vi "bigcryo_H-control.vi"(9 "Rate [T/min]":dbl=0.5, 10 "Set Field [T]":dbl, 11 "Magnet Power supply":refnum<visa-resource-name>="COM6") -> ()   [LabVIEW 2019]
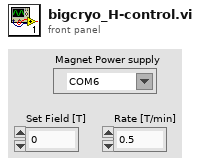
[diagram p1: front panel]
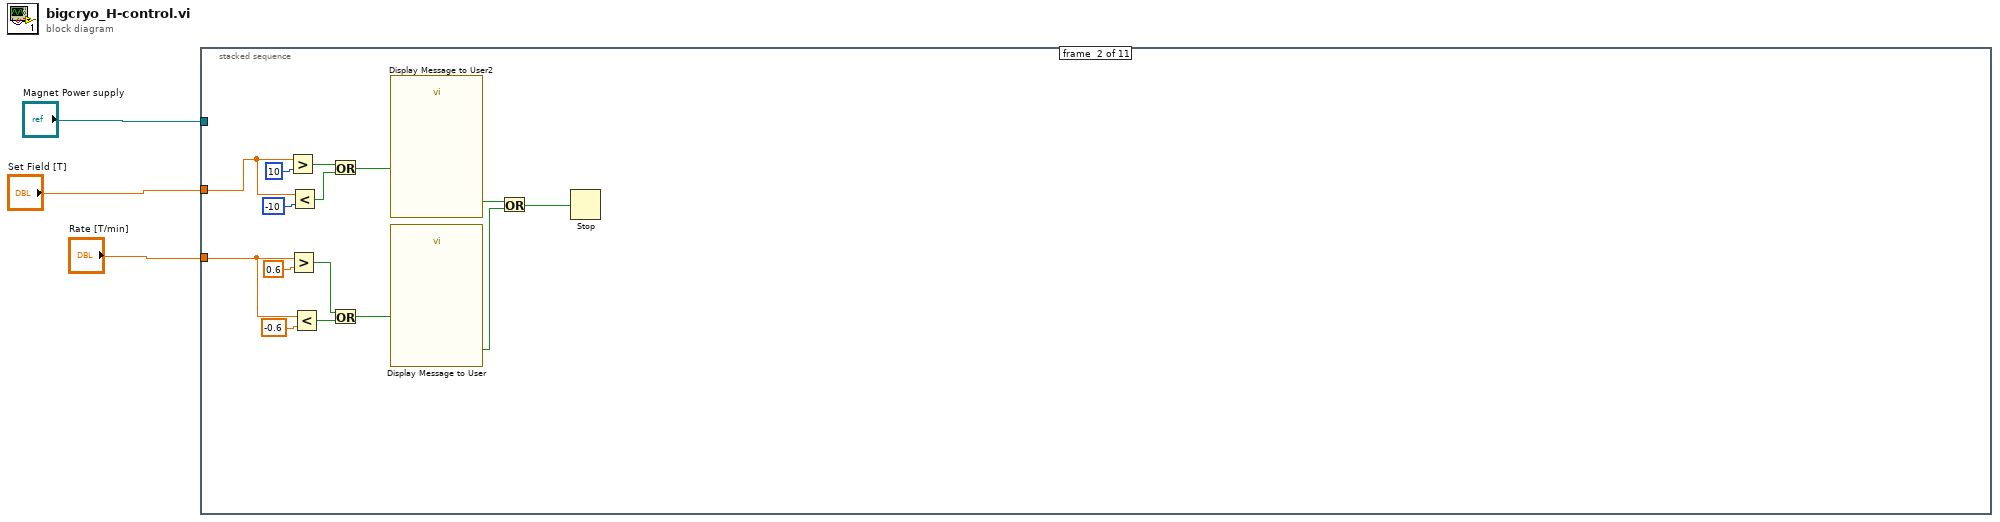
[diagram p0: block diagram]
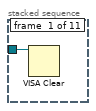
[diagram p2: hidden frame]
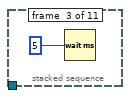
[diagram p3: hidden frame]
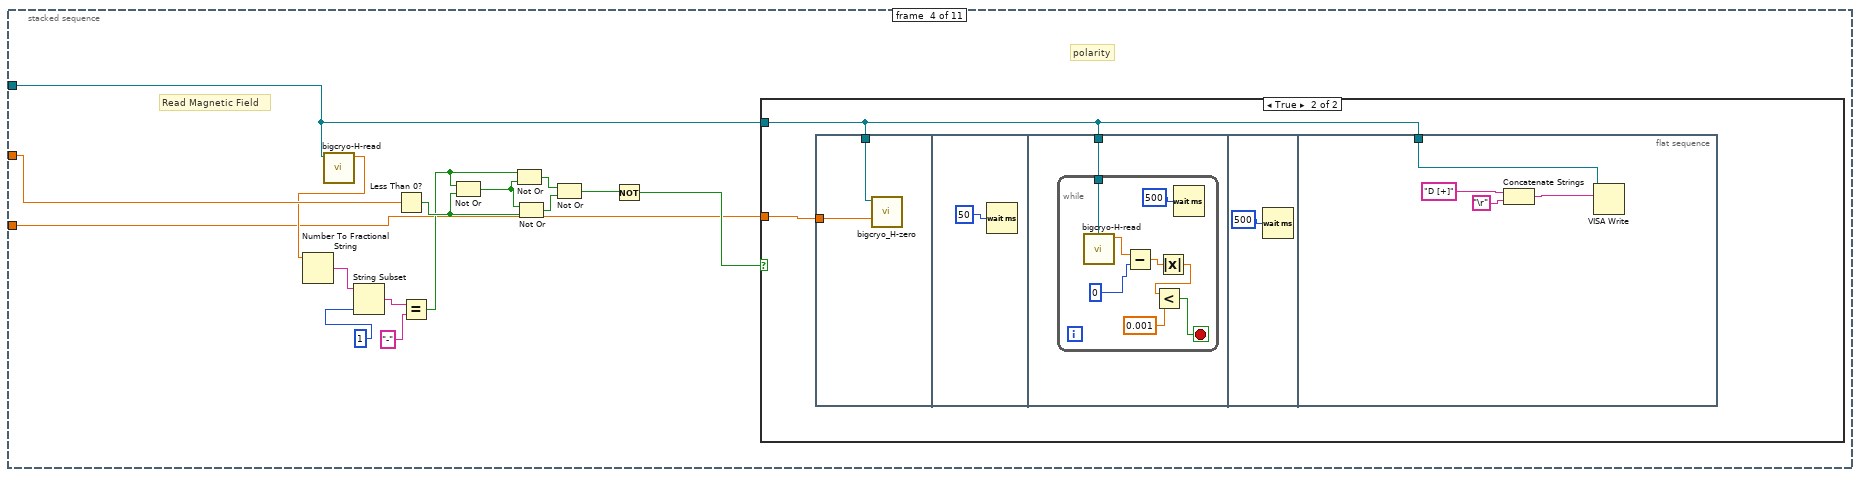
[diagram p4: hidden frame]
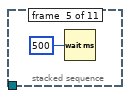
[diagram p6: hidden frame]
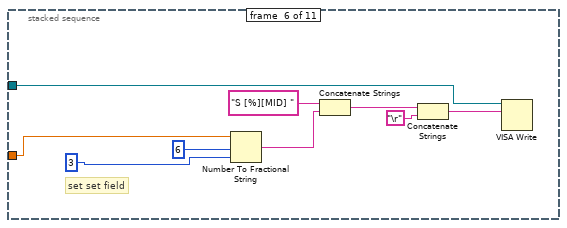
[diagram p7: hidden frame]
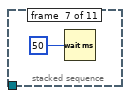
[diagram p8: hidden frame]
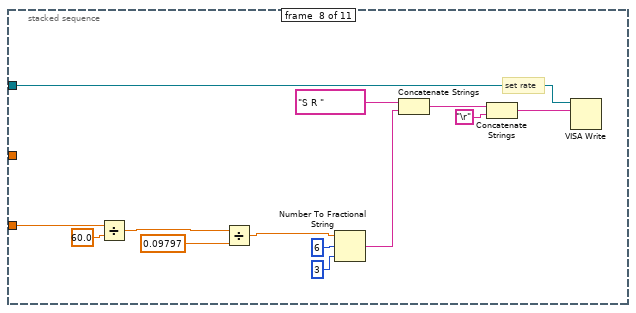
[diagram p9: hidden frame]
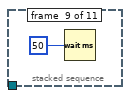
[diagram p10: hidden frame]
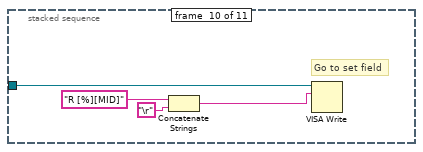
[diagram p11: hidden frame]
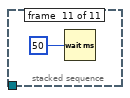
[diagram p12: hidden frame]
diagram:
  n1 = stacked-sequence {
    tunnel: "Magnet Power supply" -> [w4 _ _ w35 _ w58 _ w76 _ w81 _]
    tunnel: "Rate [T/min]" -> [_ w6 _ w21 _ _ _ w66 _ _ _]
    tunnel: "Set Field [T]" -> [_ w5 _ w34 _ w56 _ _ _ _ _]
    frame #0 {
      n2 = VISA Clear(VISA resource name=w4) -> ()  [unwired: 1 in, 2 out]
    }
    frame #1 {
      n3 = Greater?(x=w5, y=10) -> (0:w7:bool)
      n4 = Greater?(x=w6, y=0.6) -> (0:w16:bool)
      n5 = Less?(x=w5, y=-10) -> (x < y?=w12:bool)
      n6 = Less?(x=w6, y=-0.6) -> (x < y?=w15:bool)
      n7 = Or(x=w7, y=w12) -> (x .or. y?=w18:bool)
      n8 = Or(x=w16, y=w15) -> (x .or. y?=w17:bool)
      n9 = call "Display Message to User2"("Enable"=w18) -> ("OK"=w19:bool)  [unwired: 9 in, 1 out]
      n10 = call "Display Message to User"("Enable"=w17) -> ("OK"=w8:bool)  [unwired: 9 in, 1 out]
      n11 = Or(x=w19, y=w8) -> (x .or. y?=w9:bool)
      n12 = Stop(stop? (T)=w9) -> ()
    }
    frame #2 {
      n13 = Wait (ms)(milliseconds to wait=5) -> ()  [unwired: 1 out]
    }
    frame #3 {
      # "Read Magnetic Field"
      # "polarity"
      n14 = call "bigcryo-H-read.vi"("Magnet Power supply"=w35) -> ("Magnetic Field [T]"=w23:dbl)  [unwired: 9 in, 1 out]
      n15 = Number To Fractional String(number=w23) -> (F-format string=w26:string)  [unwired: 3 in]
      n16 = String Subset(string=w26, length (rest)=1 ("length (rest)")) -> (substring=w25:string)  [unwired: 1 in]
      n17 = Less Than 0?(x=w34) -> (x < 0?=w33:bool)
      n18 = Equal?(x=w25, y="-") -> (x = y?=w22:bool)
      n19 = Not Or(1:w33, 2:w22) -> (0:w32:bool)
      n20 = Not Or(1:w32, 2:w22) -> (0:w31:bool)
      n21 = Not Or(1:w33, 2:w32) -> (0:w30:bool)
      n22 = Not Or(1:w30, 2:w31) -> (0:w29:bool)
      n23 = Not(x=w29) -> (.not. x?=w28:bool)
      n24 = case shown="True" w28 {
        tunnel: w35 -> [_ w36]
        tunnel: w21 -> [_ w37]
        frame False {
        }
        frame True {
          n25 = flat-sequence {
            tunnel: w37 -> [w39]
            tunnel: w36 -> [w38]
            tunnel: w36 -> [w41]
            tunnel: w36 -> [w52]
            frame #0 {
              n26 = call "bigcryo_H-zero.vi"("Rate [T/min]"=w39, "Magnet Power supply"=w38) -> ()  [unwired: 10 in]
            }
            frame #1 {
              n27 = Wait (ms)(milliseconds to wait=50) -> ()  [unwired: 1 out]
            }
            frame #2 {
              n28 = while {
                tunnel: w41 -> [w49]
                stop <- w48 stop-if-true
                n29 = call "bigcryo-H-read.vi"("Magnet Power supply"=w49) -> ("Magnetic Field [T]"=w46:dbl)  [unwired: 9 in, 1 out]
                n30 = Subtract(x=w46, y=0) -> (x-y=w44:dbl)
                n31 = Absolute Value(x=w44) -> (abs(x)=w43:dbl)
                n32 = Less?(x=w43, y=0.001) -> (x < y?=w48:bool)
                n33 = Wait (ms)(milliseconds to wait=500) -> ()  [unwired: 1 out]
              }
            }
            frame #3 {
              n34 = Wait (ms)(milliseconds to wait=500) -> ()  [unwired: 1 out]
            }
            frame #4 {
              n35 = Concatenate Strings("D [+]" ("data"), "\r") -> (w54:string)
              n36 = VISA Write(VISA resource name=w52, write buffer=w54) -> ()  [unwired: 1 in, 3 out]
            }
          }
        }
      }
    }
    frame #4 {
      n37 = Wait (ms)(milliseconds to wait=500) -> ()  [unwired: 1 out]
    }
    frame #5 {
      # "set set field"
      n38 = Number To Fractional String(number=w56, width (-)=i16 6, precision (6)=i16 3) -> (F-format string=w61:string)  [unwired: 1 in]
      n39 = Concatenate Strings("S [%][MID] " ("string"), w61) -> (w57:string)
      n40 = Concatenate Strings(w57, "\r") -> (w60:string)
      n41 = VISA Write(VISA resource name=w58, write buffer=w60) -> ()  [unwired: 1 in, 3 out]
    }
    frame #6 {
      n42 = Wait (ms)(milliseconds to wait=50) -> ()  [unwired: 1 out]
    }
    frame #7 {
      # "set rate"
      n43 = Divide(x=w66, y=60.0) -> (x/y=w71:dbl)
      n44 = Divide(x=w71, y=0.09797) -> (x/y=w69:dbl)
      n45 = Number To Fractional String(number=w69, width (-)=i16 6, precision (6)=i16 3) -> (F-format string=w74:string)  [unwired: 1 in]
      n46 = Concatenate Strings("S R " ("string"), w74) -> (w73:string)
      n47 = Concatenate Strings(w73, "\r") -> (w78:string)
      n48 = VISA Write(VISA resource name=w76, write buffer=w78) -> ()  [unwired: 1 in, 3 out]
    }
    frame #8 {
      n49 = Wait (ms)(milliseconds to wait=50) -> ()  [unwired: 1 out]
    }
    frame #9 {
      # "Go to set field"
      n50 = Concatenate Strings("R [%][MID]" ("data"), "\r") -> (w83:string)
      n51 = VISA Write(VISA resource name=w81, write buffer=w83) -> ()  [unwired: 1 in, 3 out]
    }
    frame #10 {
      n52 = Wait (ms)(milliseconds to wait=50) -> ()  [unwired: 1 out]
    }
  }
